vi "IO_Control.vi"(3 "error in":errorcluster, 4 "btnAbort":bool=TRUE, 5 "output":refnum<k21>="Output", 6 "input":refnum<k21>="Input") -> (0 "error out":errorcluster, 1 "lightCurtain":bool, 2 "On?":bool=TRUE)   [LabVIEW 2015]
doc: "On?是否结束流程：true 运行；false 停止运行\nlightCurtain光幕触发：true 触发；false 未触发"
uses:
  <vilib>/DAQmx/read.llb/DAQmx Read (Digital 1D Bool NChan 1Samp 1Line).vi
  <vilib>/DAQmx/write.llb/DAQmx Write (Digital 1D Bool NChan 1Samp 1Line).vi
  <vilib>/DAQmx/miscellaneous.llb/DAQmx Fill In Error Info.vi
panel:
  in  "trigger":bool
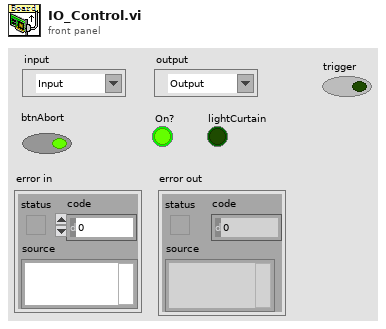
[diagram p1: front panel]
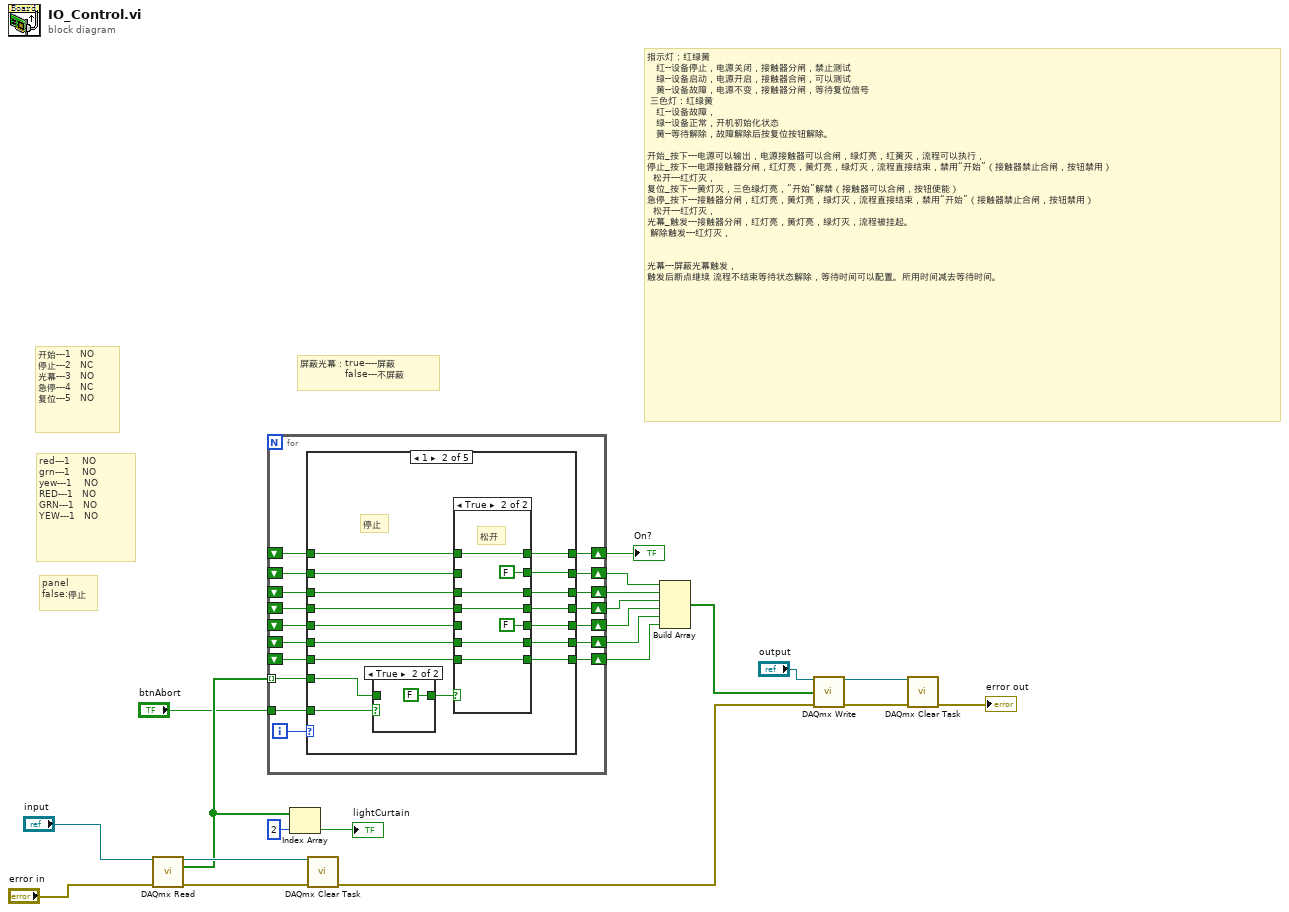
[diagram p0: block diagram]
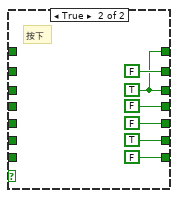
[diagram p3: hidden frame]
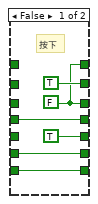
[diagram p5: hidden frame]
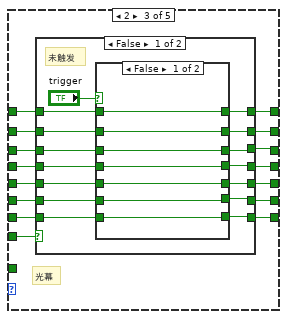
[diagram p6: hidden frame]
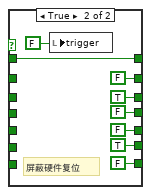
[diagram p7: hidden frame]
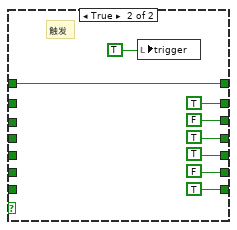
[diagram p8: hidden frame]
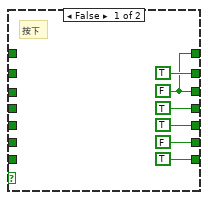
[diagram p10: hidden frame]
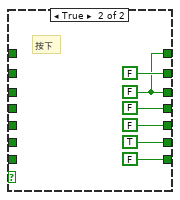
[diagram p12: hidden frame]
diagram:
  # "panel\nfalse:停止"
  # "屏蔽光幕：true----屏蔽\n               false---不屏蔽"
  # "指示灯：红绿黄\n\t\t\t红--设备停止，电源关闭，接触器分闸，禁止测试\n\t\t\t绿--设备启动，电源开启，接触器合闸，可以测试\n\t\t\t黄--设备故障，电源不变，接触器分闸，等待复位信号\n\t三色灯：红绿黄\n\t\t\t红--设备故障，\n\t\t\t绿--设备正常，开机初始化状态\n\t\t\t黄--等待解除，故障解除后按复位按钮解除。\n\n开始_按下---电源可以输出，电源接触器可以合闸，绿灯亮，红黄灭，流程可以执行，\n停止_按下---电源接触器分闸，红灯亮，黄灯亮，绿灯灭，流程直接结束，禁用“开始”（接触器禁止合闸，按钮禁用）\n\t 松开---红灯灭，\n复位_按下---黄灯灭，三色绿灯亮，“开始”解禁（接触器可以合闸，按钮使能）\n急停_按下---接触器分闸，红灯亮，黄灯亮，绿灯灭，流程直接结束，禁用“开始”（接触器禁止合闸，按钮禁用）\n\t 松开---红灯灭，\n光幕_触发---接触器分闸，红灯亮，黄灯亮，绿灯灭，流程被挂起。\n 解除触发---红灯灭，\n\n\n光幕---屏蔽光幕触发，\n触发后断点继续 流程不结束等待状态解除，等待时间可以配置。所用时间减去等待时间。"
  # "red---1    NO \ngrn---1    NO\nyew---1    NO\nRED---1   NO\nGRN---1   NO\nYEW---1   NO"
  # "开始---1   NO \n停止---2   NC\n光幕---3   NO\n急停---4   NC\n复位---5   NO"
  n1 = call-poly <vilib>:"DAQmx Read.vi"("task/channels in"="input", "error in"="error in") -> ("task out"=w11:refnum<k21>, "data"=w7:bool[], "error out"=w10:errorcluster)  [unwired: 11 in]
  n2 = for {
    shift-right: [w37] -> w21
    shift-left: _ -> [w36]
    shift-right: [w34] -> w19
    shift-left: _ -> [w29]
    shift-right: [w33] -> w18
    shift-left: _ -> [w28]
    shift-right: [w32] -> w17
    shift-left: _ -> [w27]
    shift-right: [w31] -> w16
    shift-left: _ -> [w26]
    shift-right: [w30] -> w15
    shift-left: _ -> [w25]
    shift-right: [w35] -> w20
    shift-left: _ -> [w24]
    tunnel: w7 -> [w23] mode=indexing
    tunnel: "btnAbort" -> [w22]
    i -> [w38]
    n3 = case shown="1" w38 {
      tunnel: [w53 w82 w112 w166 w194] -> w37
      tunnel: w36 -> [w52 w75 w105 w153 w188]
      tunnel: [w51 w77 w107 w160 w182] -> w35
      tunnel: [w50 w81 w111 w165 w193] -> w34
      tunnel: [w49 w80 w110 w161 w192] -> w33
      tunnel: [w48 w79 w109 w162 w191] -> w32
      tunnel: [w47 w78 w108 w163 w190] -> w31
      tunnel: [w46 w83 w113 w164 w189] -> w30
      tunnel: w29 -> [w45 w74 w104 w158 w187]
      tunnel: w28 -> [w44 w73 w103 w157 w186]
      tunnel: w27 -> [w43 w72 w102 w152 w185]
      tunnel: w26 -> [w42 w71 w101 w156 w184]
      tunnel: w25 -> [w41 w70 w100 w155 w183]
      tunnel: w24 -> [w40 w76 w106 w159 w181]
      tunnel: w23 -> [w39 w69 w99 w154 w180]
      tunnel: w22 -> [_ w67 _ _ _]
      frame 0, Default {
        # "开始"
        n4 = case shown="False" w39 {
          tunnel: [w60 FALSE] -> w53
          tunnel: w52 -> [w60 _]
          tunnel: [w54 w61] -> w51
          tunnel: [w59 w61] -> w50
          tunnel: [w58 FALSE] -> w49
          tunnel: [w57 FALSE] -> w48
          tunnel: [w56 TRUE] -> w47
          tunnel: [w55 FALSE] -> w46
          tunnel: w45 -> [w59 _]
          tunnel: w44 -> [w58 _]
          tunnel: w43 -> [w57 _]
          tunnel: w42 -> [w56 _]
          tunnel: w41 -> [w55 _]
          tunnel: w40 -> [w54 _]
          frame False {
            # "松开"
          }
          frame True {
            w61 = TRUE
            # "按下"
          }
        }
      }
      frame 1 {
        # "停止"
        n5 = case shown="True" w67 {
          tunnel: [w84 FALSE ("Boolean")] -> w68
          tunnel: w69 -> [w84 _]
          frame False {
          }
          frame True {
          }
        }
        n6 = case shown="True" w68 {
          tunnel: [w88 w94] -> w83
          tunnel: [TRUE FALSE] -> w82
          tunnel: [w89 w97] -> w81
          tunnel: [w87 w96] -> w80
          tunnel: [TRUE FALSE] -> w79
          tunnel: [w86 w95] -> w78
          tunnel: [w89 w98] -> w77
          tunnel: w76 -> [_ w98]
          tunnel: w75 -> [_ _]
          tunnel: w74 -> [_ w97]
          tunnel: w73 -> [w87 w96]
          tunnel: w72 -> [_ _]
          tunnel: w71 -> [w86 w95]
          tunnel: w70 -> [w88 w94]
          frame False {
            w89 = FALSE
            # "按下"
          }
          frame True {
            # "松开"
          }
        }
      }
      frame 2 {
        # "光幕"
        n7 = case shown="False" w99 {
          tunnel: [w115 TRUE] -> w113
          tunnel: [w120 TRUE] -> w112
          tunnel: [w119 FALSE] -> w111
          tunnel: [w118 TRUE] -> w110
          tunnel: [w117 TRUE] -> w109
          tunnel: [w116 FALSE] -> w108
          tunnel: [w121 w144] -> w107
          tunnel: w106 -> [w128 w144]
          tunnel: w105 -> [w127 _]
          tunnel: w104 -> [w126 _]
          tunnel: w103 -> [w125 _]
          tunnel: w102 -> [w124 _]
          tunnel: w101 -> [w123 _]
          tunnel: w100 -> [w122 _]
          frame False {
            # "未触发"
            n8 = case shown="False" "trigger" {
              tunnel: w128 -> [w134 w136]
              tunnel: [w135 FALSE] -> w120
              tunnel: w127 -> [w135 _]
              tunnel: [w134 w136] -> w121
              tunnel: [w133 TRUE] -> w119
              tunnel: w126 -> [w133 _]
              tunnel: [w132 FALSE] -> w118
              tunnel: w125 -> [w132 _]
              tunnel: [w131 FALSE] -> w117
              tunnel: w124 -> [w131 _]
              tunnel: [w130 TRUE] -> w116
              tunnel: w123 -> [w130 _]
              tunnel: [w129 FALSE] -> w115
              tunnel: w122 -> [w129 _]
              frame False {
              }
              frame True {
                # "屏蔽硬件复位"
                n9 = local write "trigger"(FALSE ("trigger")) -> ()
              }
            }
          }
          frame True {
            # "触发"
            n10 = local write "trigger"(TRUE ("trigger")) -> ()
          }
        }
      }
      frame 3 {
        # "急停"
        n11 = case shown="True" w154 {
          tunnel: [TRUE w174] -> w166
          tunnel: [w167 w178] -> w165
          tunnel: [TRUE w175] -> w164
          tunnel: [FALSE w176] -> w163
          tunnel: [TRUE w173] -> w162
          tunnel: [TRUE w177] -> w161
          tunnel: [w167 w179] -> w160
          tunnel: w159 -> [_ w179]
          tunnel: w158 -> [_ w178]
          tunnel: w157 -> [_ w177]
          tunnel: w156 -> [_ w176]
          tunnel: w155 -> [_ w175]
          tunnel: w153 -> [_ w174]
          tunnel: w152 -> [_ w173]
          frame False {
            w167 = FALSE
            # "按下"
          }
          frame True {
            # "松开"
          }
        }
      }
      frame 4 {
        # "复位"
        n12 = case shown="False" w180 {
          tunnel: [w201 FALSE] -> w194
          tunnel: [w200 w202] -> w193
          tunnel: [w199 FALSE] -> w192
          tunnel: [w198 FALSE] -> w191
          tunnel: [w197 TRUE] -> w190
          tunnel: [w196 FALSE] -> w189
          tunnel: w188 -> [w201 _]
          tunnel: w187 -> [w200 _]
          tunnel: w186 -> [w199 _]
          tunnel: w185 -> [w198 _]
          tunnel: w184 -> [w197 _]
          tunnel: w183 -> [w196 _]
          tunnel: [w195 w202] -> w182
          tunnel: w181 -> [w195 _]
          frame False {
            # "松开"
          }
          frame True {
            w202 = FALSE
            # "按下"
          }
        }
      }
    }
  }
  "On?" <- w20
  n13 = Index Array(array=w7, index=2) -> (element=→"lightCurtain":bool)
  n14 = call <vilib>:"DAQmx Clear Task.vi"("task in"=w11, "error in"=w10) -> ("error out"=w9:errorcluster)  [unwired: 13 in]
  n15 = Build Array(w21, w19, w18, w17, w16, w15) -> (w14:bool[])
  n16 = call-poly <vilib>:"DAQmx Write.vi"("task/channels in"="output", "data"=w14, "error in"=w9) -> ("task out"=w1:refnum<k21>, "error out"=w3:errorcluster)  [unwired: 10 in, 1 out]
  n17 = call <vilib>:"DAQmx Clear Task.vi"("task in"=w1, "error in"=w3) -> ("error out"=→"error out":errorcluster)  [unwired: 13 in]
